vi "Duplicate Config check.vi"(10 "Data in":T1(array[cluster])) -> (2 "Channel list indication":bool)   [LabVIEW 2020]
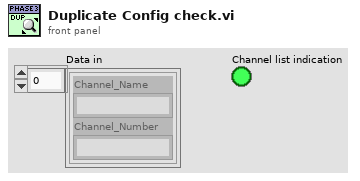
[diagram p1: front panel]
types:
  T1 = cluster{"Channel_Name":string, "Channel_Number":string}[]
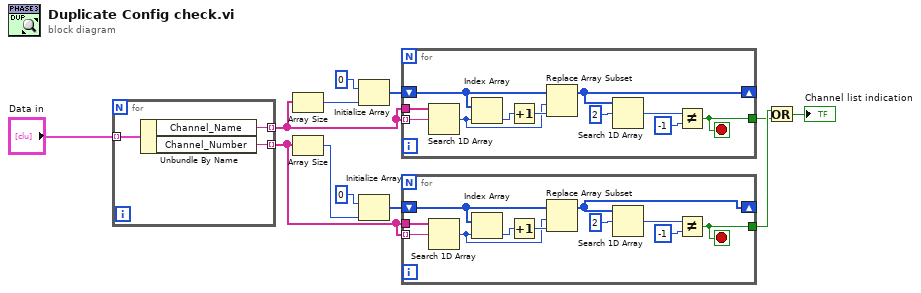
[diagram p0: block diagram]
diagram:
  n1 = for {
    tunnel: [w15] -> w9 mode=indexing
    tunnel: [w14] -> w5 mode=indexing
    tunnel: "Data in" -> [w13] mode=indexing
    n2 = Unbundle By Name(w13) -> ("Channel_Name"=w15:string, "Channel_Number"=w14:string)
  }
  n3 = Array Size(array=w9) -> (size(s)=w10:i32)
  n4 = Array Size(array=w5) -> (size(s)=w8:i32)
  n5 = Initialize Array(u32 0 ("element"), w10) -> (w12:u32[])
  n6 = Initialize Array(u32 0 ("element"), w8) -> (w6:u32[])
  n7 = for {
    tunnel: w9 -> [w25] mode=indexing
    tunnel: w9 -> [w26]
    shift-right: [w20] -> _
    shift-left: w12 -> [w24]
    tunnel: [w16] -> w3
    stop <- w16 stop-if-true
    n8 = Search 1D Array(1D array=w26, element=w25) -> (index of element=w21:i32)  [unwired: 1 in]
    n9 = Index Array(array=w24, index=w21) -> (element=w23:u32)
    n10 = Increment(x=w23) -> (x+1=w22:u32)
    n11 = Replace Array Subset(array=w24, new element=w22, index=w21) -> (w20:u32[])
    n12 = Search 1D Array(1D array=w20, element=u32 2) -> (index of element=w18:i32)  [unwired: 1 in]
    n13 = Not Equal?(x=w18, y=-1) -> (x != y?=w16:bool)
  }
  n14 = for {
    tunnel: w5 -> [w36] mode=indexing
    tunnel: w5 -> [w37]
    shift-right: [w31] -> _
    shift-left: w6 -> [w35]
    tunnel: [w27] -> w4
    stop <- w27 stop-if-true
    n15 = Search 1D Array(1D array=w37, element=w36) -> (index of element=w32:i32)  [unwired: 1 in]
    n16 = Index Array(array=w35, index=w32) -> (element=w34:u32)
    n17 = Increment(x=w34) -> (x+1=w33:u32)
    n18 = Replace Array Subset(array=w35, new element=w33, index=w32) -> (w31:u32[])
    n19 = Search 1D Array(1D array=w31, element=u32 2) -> (index of element=w29:i32)  [unwired: 1 in]
    n20 = Not Equal?(x=w29, y=-1) -> (x != y?=w27:bool)
  }
  n21 = Or(x=w4, y=w3) -> (x .or. y?=→"Channel list indication":bool)
